vi "Tbl_filter.vi"(7 "Sort type":u16(ring) items=["Numeric", "Alpha"], 10 "Col to sort":i32) -> (3 "Table out":i32[](listbox), 11 "Table in":i32[](listbox))   [LabVIEW 2017]
uses:
  71f7bdd7-b5bf-4e11-9e2b-918d328992ce.vi
  <vilib>/Array/Sort 2D Array - Pop Stack.vi
  <vilib>/Array/Sort 2D Array - Push Stack.vi
  <vilib>/Analysis/NI_AALPro.lvlib
panel:
  in  "Active Cell:Cell Justification":enum16{"Left", "Center", "Right"}(ring)
  out "Justify arr 2":enum16{"Left", "Center", "Right"}[](array[ring])
  out "Justify arr":enum16{"Left", "Center", "Right"}[](array[ring])
  out "File size (KB)":dbl[](array[numeric])
  out "Sorted Index":i32[](array[numeric])
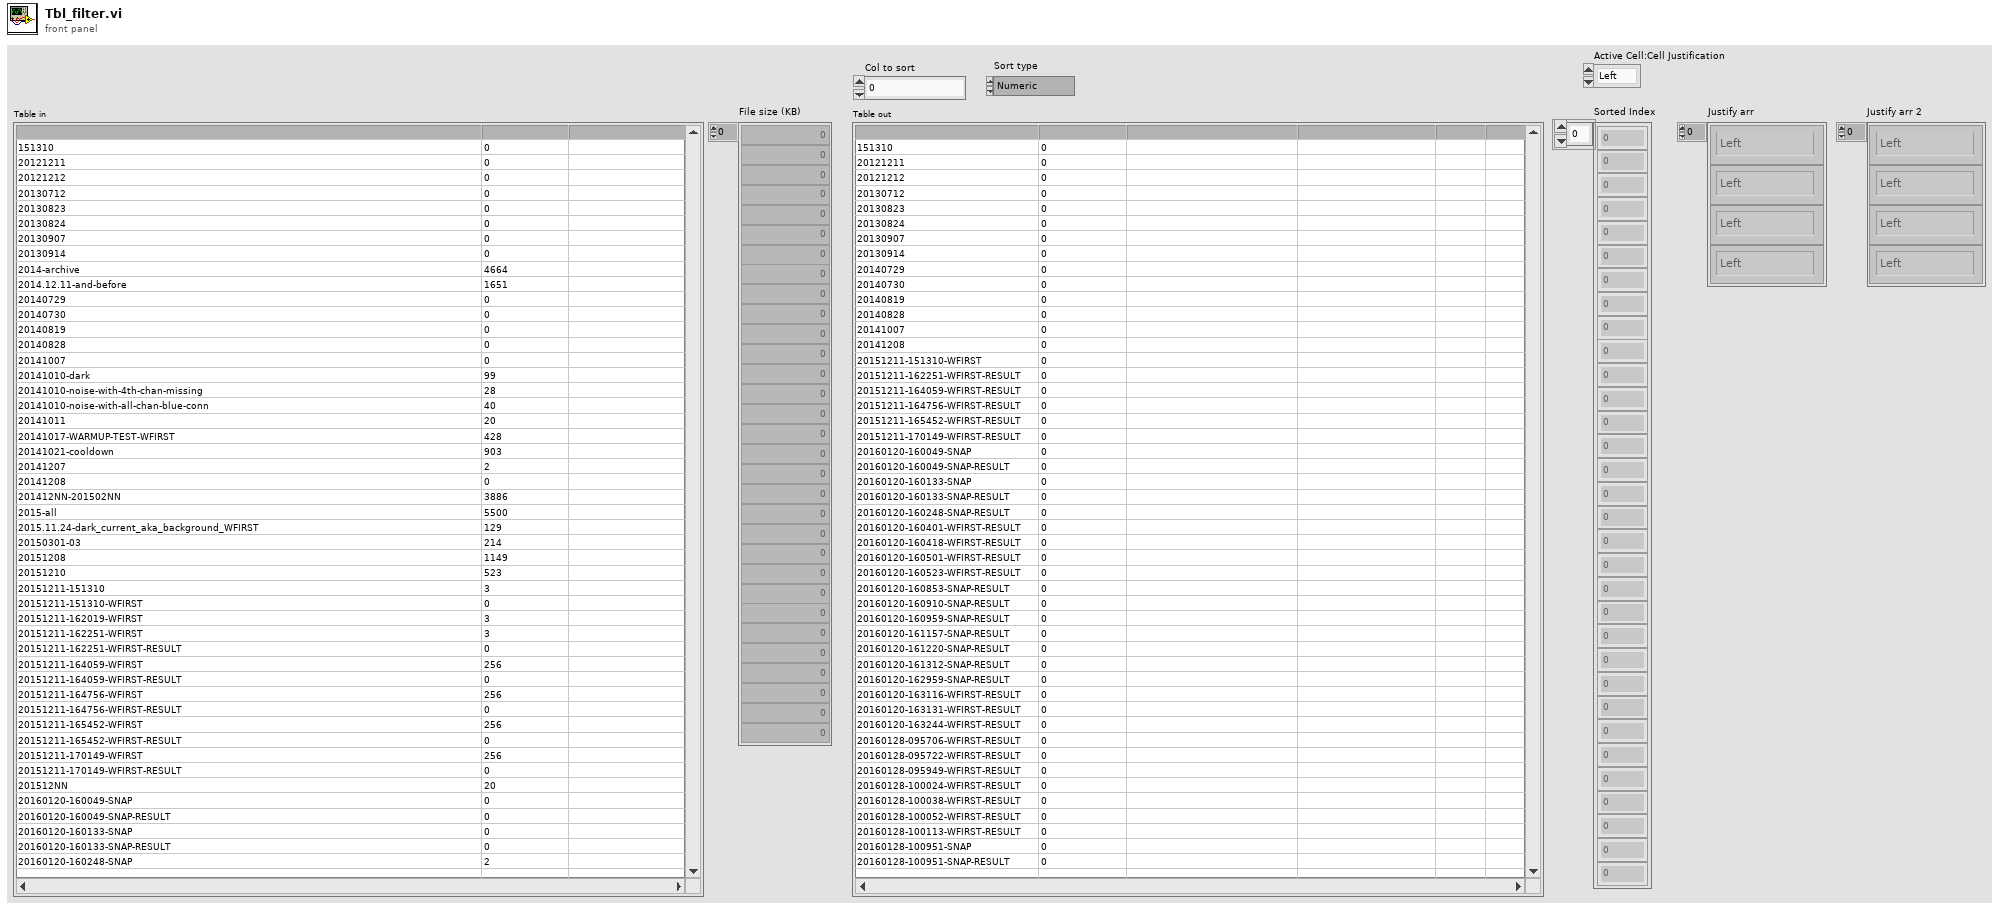
[diagram p1: front panel]
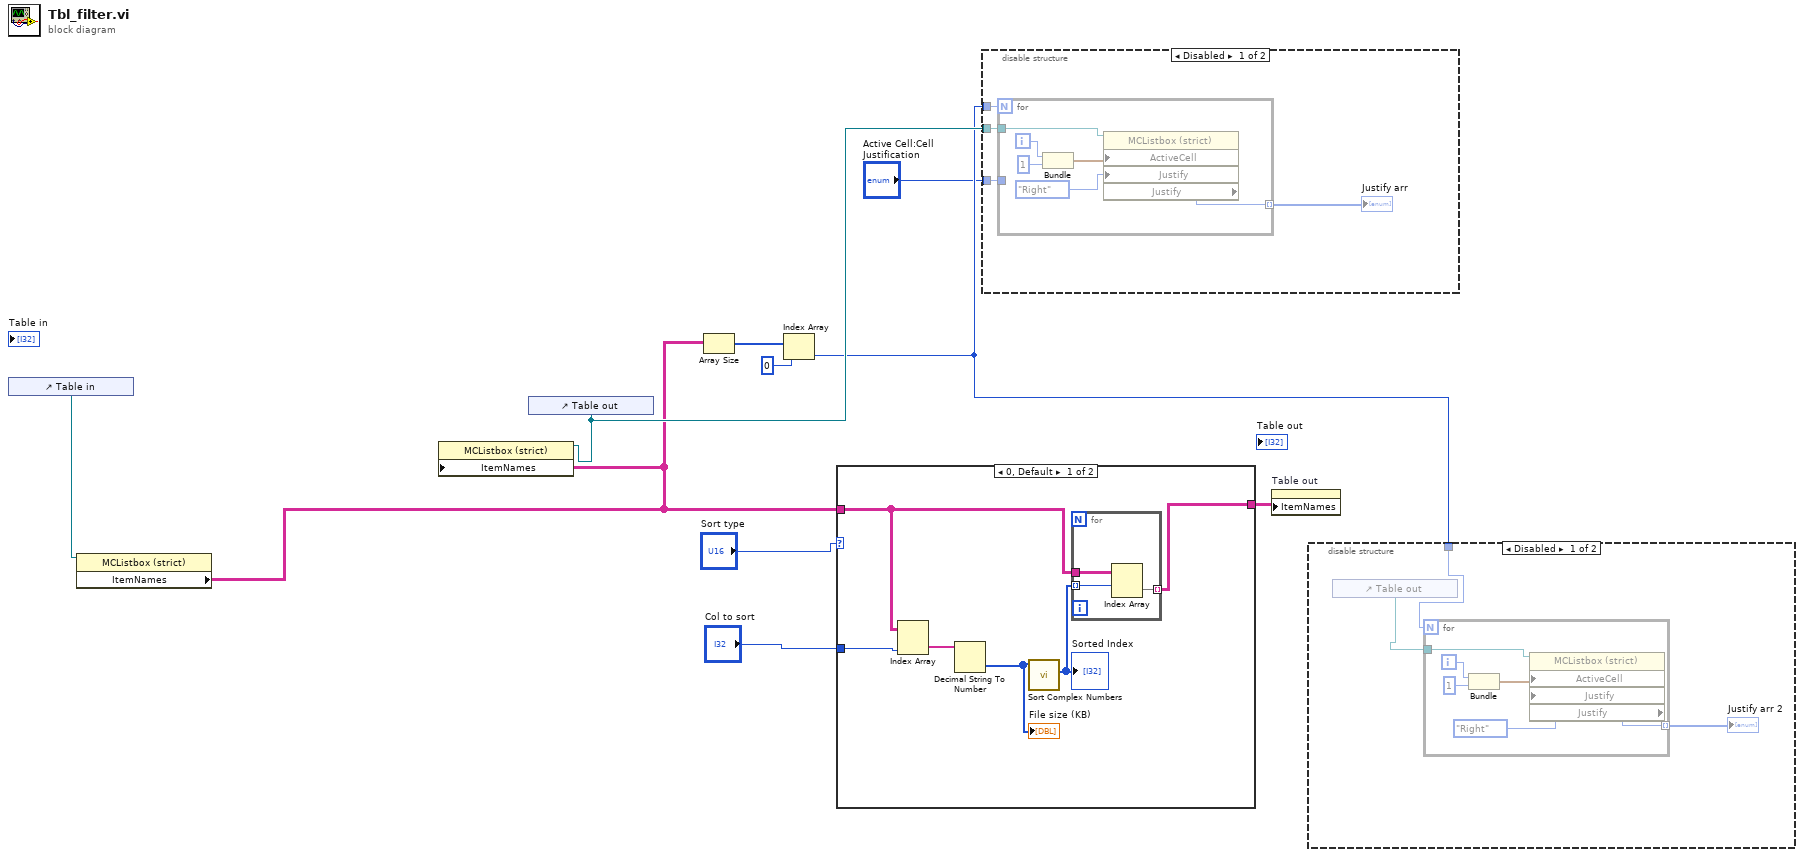
[diagram p0: block diagram]
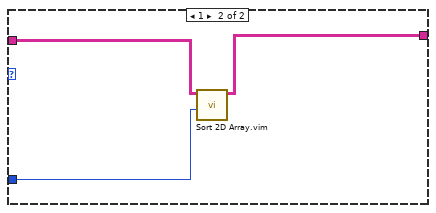
[diagram p4: hidden frame]
diagram:
  n1 = control-ref of="Table in"() -> (w10:refnum<vi>)
  n2 = property on="Property Node" class="MCListbox (strict)"(reference=w10) -> ("ItemNames"=w6:string[][])  [unwired: 1 in, 2 out]
  n3 = control-ref of="Table out"() -> (w9:refnum<vi>)
  n4 = property on="Property Node" class="MCListbox (strict)"(reference=w9, "ItemNames"=w6) -> ()  [unwired: 1 in, 2 out]
  n5 = Array Size(array=w6) -> (size(s)=w8:i32[])
  n6 = Index Array(array=w8, index=0) -> (element=w2:i32)
  n7 = case shown="0, Default" "Sort type" {
    tunnel: w6 -> [w11 w22]
    tunnel: "Col to sort" -> [w13 w21]
    tunnel: [w12 w20] -> w3
    frame 0, Default {
      n8 = Index Array(array=w11, index (col)=w13) -> (element=w16:string[])  [unwired: 1 in]
      n9 = Decimal String To Number(string=w16) -> (number=w15:i32[])  [unwired: 2 in, 1 out]
      "File size (KB)" <- w15
      n10 = call <vilib>:"Sort Complex Numbers.vi"("Complex Numbers"=w15) -> ("Sorted Index"=w14:i32[])  [unwired: 8 in, 2 out]
      "Sorted Index" <- w14
      n11 = for {
        tunnel: w11 -> [w19]
        tunnel: w14 -> [w18] mode=indexing
        tunnel: [w17] -> w12 mode=indexing
        n12 = Index Array(array=w19, index (row)=w18) -> (element=w17:string[])  [unwired: 1 in]
      }
    }
    frame 1 {
      n13 = call "Sort 2D Array.vim"("index"=w21, "2D array"=w22) -> ("sorted 2D array"=w20:string[][])  [unwired: 8 in, 1 out]
    }
  }
  n14 = disable-structure shown="Disabled" {
    disable-tunnel: w9 -> [w25 _]
    disable-tunnel: w2 -> [w24 _]
    disable-tunnel: "Active Cell:Cell Justification" -> [w23 _]
    frame Disabled {
      n15 = for {
        N: w24 -> [_]
        tunnel: [w29] -> w26 mode=indexing
        tunnel: w25 -> [w28]
        tunnel: w23 -> [_]
        i -> [w31]
        n16 = Bundle(w31, "Column"=1) -> (w32:cluster{i32, "Column":i32})  [unwired: 1 in]
        n17 = property on="Property Node" class="MCListbox (strict)"(reference=w28, "ActiveCell"=w32, "Justify"=enum16{"Left", "Center", "Right"}."Right" ("Active Cell:Cell Justification")) -> ("Justify"=w29:enum16{"Left", "Center", "Right"})  [unwired: 1 in, 2 out]
      }
      "Justify arr" <- w26
    }
    frame Enabled {
    }
  }
  n18 = property on="Table out" class="MCListbox (strict)"("ItemNames"=w3) -> ()  [unwired: 2 in, 2 out]
  n19 = disable-structure shown="Disabled" {
    disable-tunnel: w2 -> [w33 _]
    frame Disabled {
      n20 = control-ref of="Table out"() -> (w34:refnum<vi>)
      n21 = for {
        N: w33 -> [_]
        tunnel: [w38] -> w35 mode=indexing
        tunnel: w34 -> [w36]
        i -> [w40]
        n22 = Bundle(w40, "Column"=1) -> (w41:cluster{i32, "Column":i32})  [unwired: 1 in]
        n23 = property on="Property Node" class="MCListbox (strict)"(reference=w36, "ActiveCell"=w41, "Justify"=enum16{"Left", "Center", "Right"}."Right" ("Active Cell:Cell Justification")) -> ("Justify"=w38:enum16{"Left", "Center", "Right"})  [unwired: 1 in, 2 out]
      }
      "Justify arr 2" <- w35
    }
    frame Enabled {
    }
  }
